vi "Parse Data Packet for Writing.vi"(10 "First Log Value in":bool, 11 "WiBCI16T Data in":T1 {"Reg Map"."ADS2" format="%x"; "Reg Map"."ADS1" format="%x"}) -> (3 "Array":dbl[](array[numeric]))   [LabVIEW 2016, in "Logger.lvlib"]
uses:
  Logger.lvlib
  Acquisition/WiBCI16T_Data.ctl
  Acquisition/WiBCI16T_Status.ctl
  Acquisition/Reg_Map.ctl
  Acquisition/Acquisition.lvlib
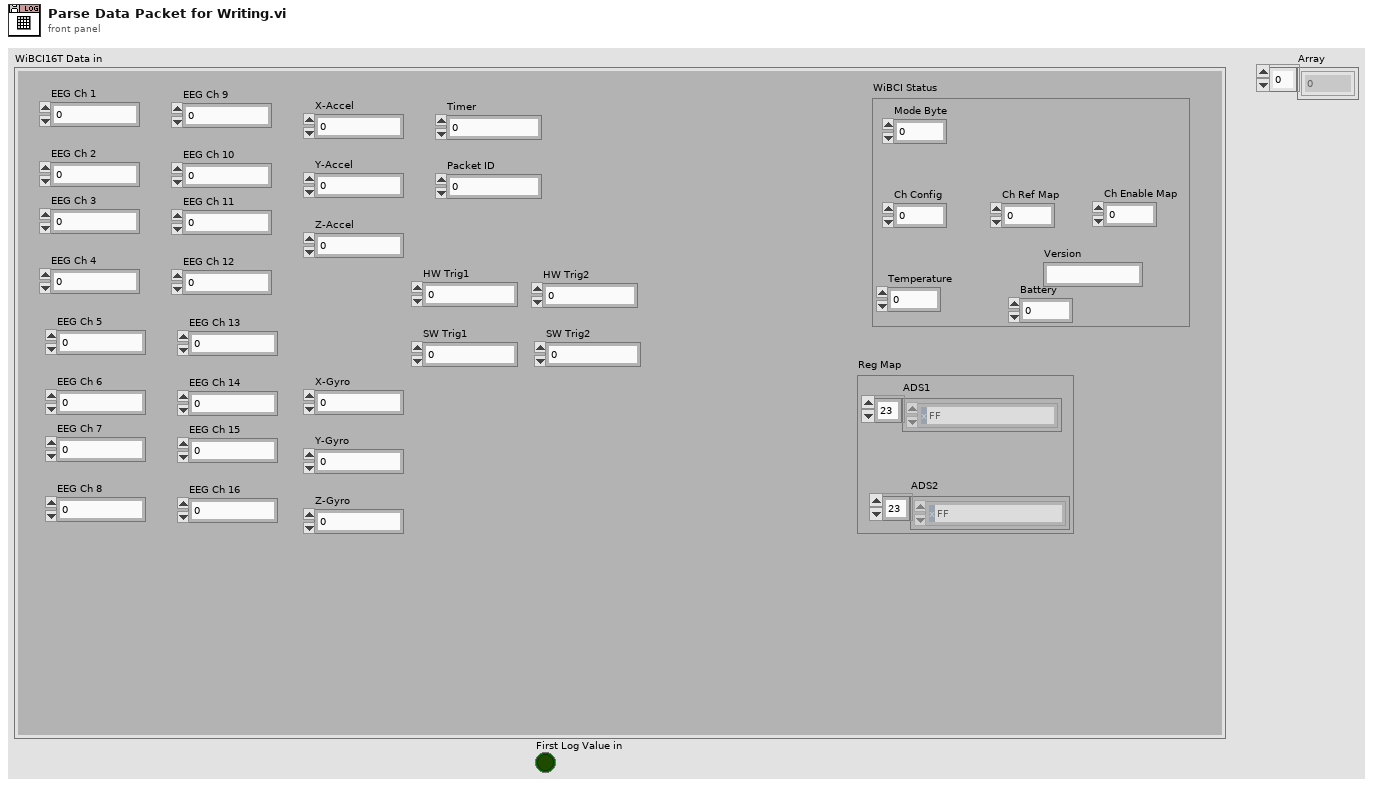
[diagram p1: front panel]
types:
  T1 = typedef "Acquisition.lvlib/WiBCI16T_Data.ctl" = cluster{"EEG Ch 1":dbl, "EEG Ch 2":dbl, "EEG Ch 3":dbl, "EEG Ch 4":dbl, "EEG Ch 5":dbl, "EEG Ch 6":dbl, "EEG Ch 7":dbl, "EEG Ch 8":dbl, "EEG Ch 9":dbl, "EEG Ch 10":dbl, "EEG Ch 11":dbl, "EEG Ch 12":dbl, "EEG Ch 13":dbl, "EEG Ch 14":dbl, "EEG Ch 15":dbl, "EEG Ch 16":dbl, "X-Accel":i16, "Y-Accel":i16, "Z-Accel":i16, "X-Gyro":i16, "Y-Gyro":i16, "Z-Gyro":i16, "Timer":u32, "Packet ID":u32, "HW Trig1":u8, "SW Trig1":i8, "HW Trig2":u8, "SW Trig2":i8, "WiBCI Status":T2, "Reg Map":T3}
  T2 = typedef "Acquisition.lvlib/WiBCI16T_Status.ctl" = cluster{"Mode Byte":u8, "Ch Config":u8, "Ch Ref Map":u16, "Ch Enable Map":u16, "Temperature":sgl, "Battery":u8, "Version":string}
  T3 = typedef "Acquisition.lvlib/Reg_Map.ctl" = cluster{"ADS1":u8[], "ADS2":u8[]}
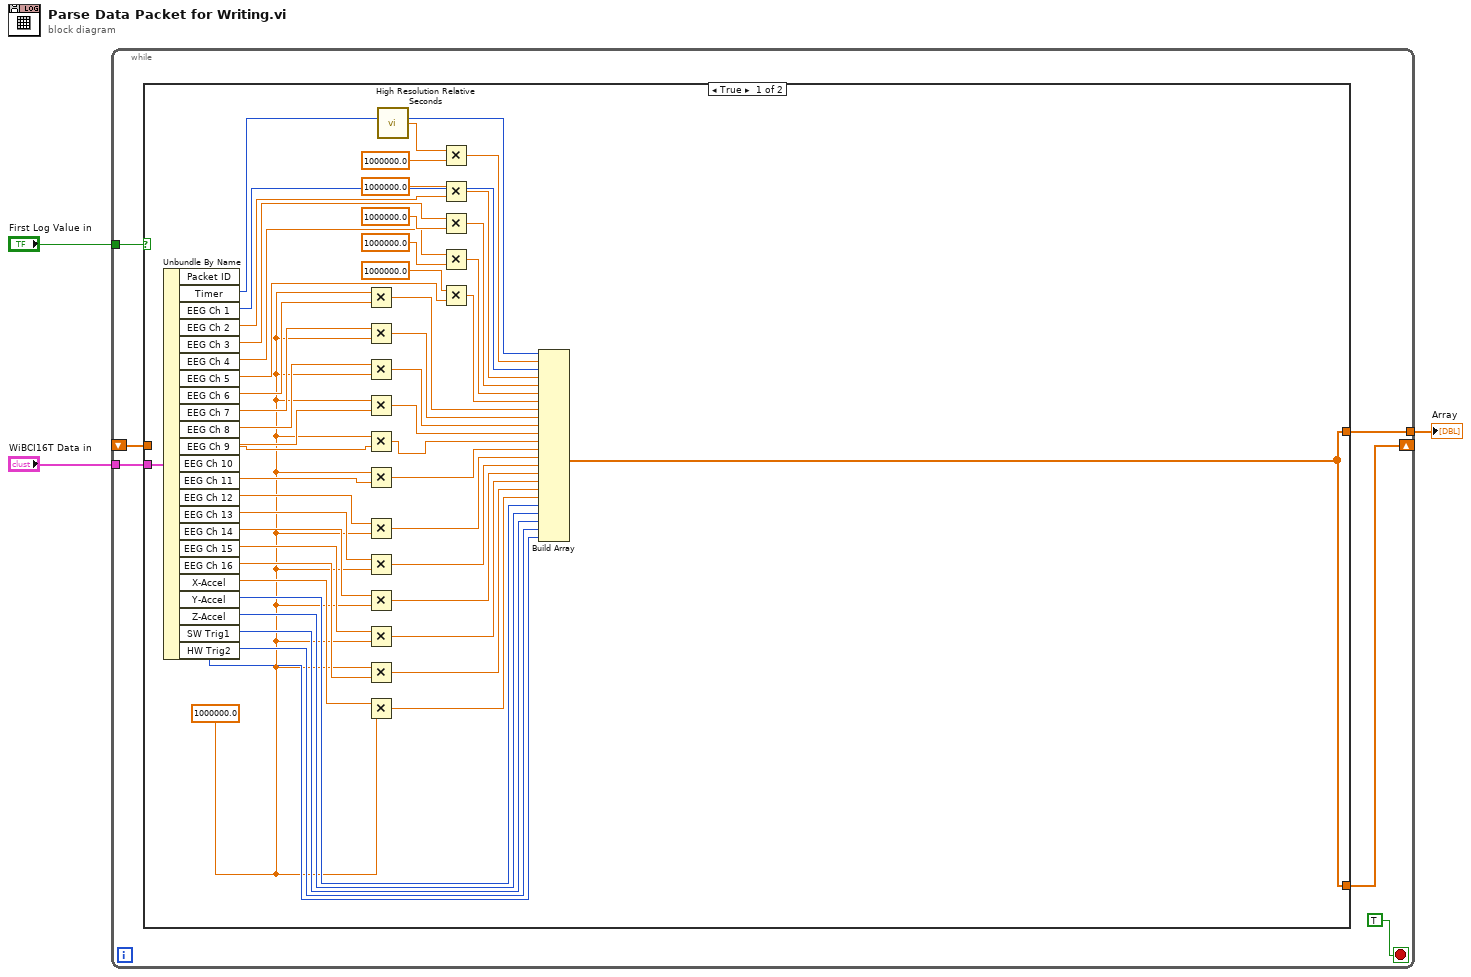
[diagram p0: block diagram]
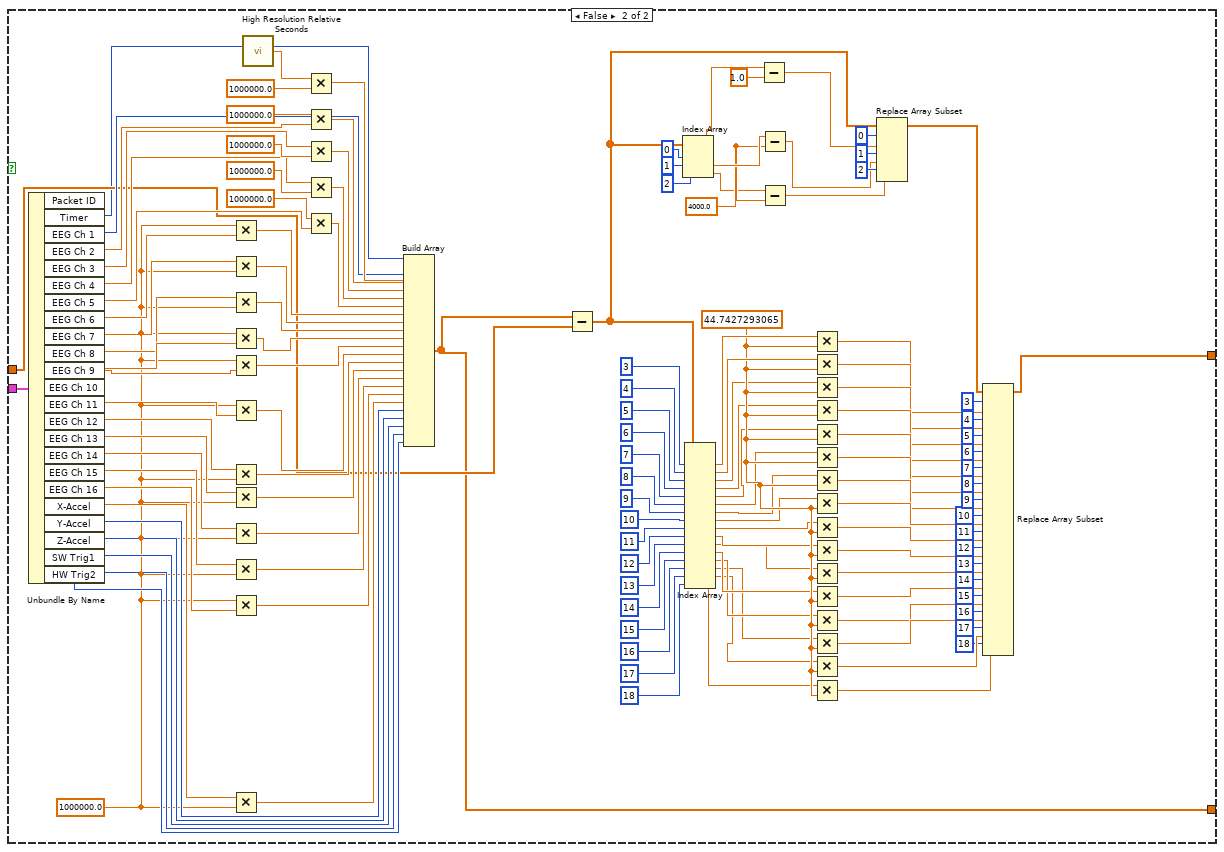
[diagram p2: hidden frame]
diagram:
  n1 = while {
    tunnel: [w9] -> w3
    shift-right: [w5] -> _
    shift-left: _ -> [w8]
    tunnel: "First Log Value in" -> [w6]
    tunnel: "WiBCI16T Data in" -> [w4]
    stop <- TRUE stop-if-true
    n2 = case shown="True" w6 {
      tunnel: [w10 w75] -> w9
      tunnel: w8 -> [_ w143]
      tunnel: [w10 w142] -> w5
      tunnel: w4 -> [w11 w144]
      frame True {
        w12 = 1000000.0 ("x")
        n3 = Unbundle By Name(w11) -> ("Packet ID"=w29:u32, "Timer"=w31:u32, "EEG Ch 1"=w32:dbl, "EEG Ch 2"=w33:dbl, "EEG Ch 3"=w34:dbl, "EEG Ch 4"=w35:dbl, "EEG Ch 5"=w36:dbl, "EEG Ch 6"=w37:dbl, "EEG Ch 7"=w38:dbl, "EEG Ch 8"=w39:dbl, "EEG Ch 9"=w40:dbl, "EEG Ch 10"=w41:dbl, "EEG Ch 11"=w42:dbl, "EEG Ch 12"=w43:dbl, "EEG Ch 13"=w44:dbl, "EEG Ch 14"=w45:dbl, "EEG Ch 15"=w46:dbl, "EEG Ch 16"=w47:dbl, "X-Accel"=w48:i16, "Y-Accel"=w49:i16, "Z-Accel"=w50:i16, "SW Trig1"=w51:i8, "HW Trig2"=w52:u8)
        n4 = Multiply(x=w12, y=w36) -> (x*y=w24:dbl)
        n5 = Multiply(x=w37, y=w12) -> (x*y=w23:dbl)
        n6 = Multiply(x=w38, y=w12) -> (x*y=w22:dbl)
        n7 = Multiply(x=w12, y=w39) -> (x*y=w21:dbl)
        n8 = Multiply(x=w12, y=w40) -> (x*y=w20:dbl)
        n9 = Multiply(x=w12, y=w41) -> (x*y=w19:dbl)
        n10 = Multiply(x=w42, y=w12) -> (x*y=w18:dbl)
        n11 = Multiply(x=w43, y=w12) -> (x*y=w17:dbl)
        n12 = Multiply(x=w44, y=w12) -> (x*y=w16:dbl)
        n13 = Multiply(x=w45, y=w12) -> (x*y=w14:dbl)
        n14 = Multiply(x=w12, y=w46) -> (x*y=w15:dbl)
        n15 = Multiply(x=w47, y=w12) -> (x*y=w13:dbl)
        n16 = call <vilib>:"High Resolution Relative Seconds.vi"() -> ("relative seconds"=w30:dbl)
        n17 = Multiply(x=w30, y=1000000.0) -> (x*y=w53:dbl)
        n18 = Multiply(x=1000000.0, y=w32) -> (x*y=w55:dbl)
        n19 = Multiply(x=w33, y=1000000.0) -> (x*y=w57:dbl)
        n20 = Multiply(x=w34, y=1000000.0) -> (x*y=w28:dbl)
        n21 = Multiply(x=1000000.0, y=w35) -> (x*y=w26:dbl)
        n22 = Build Array(w29, w53, w31, w55, w57, w28, w26, w24, w23, w22, w21, w20, w19, w18, w17, w16, w14, w15, w13, w48, w49, w50, w51, w52) -> (w10:dbl[])
      }
      frame False {
        w108 = 44.7427293065
        w137 = 4000.0 ("y")
        w145 = 1000000.0 ("x")
        n23 = Unbundle By Name(w144) -> ("Packet ID"=w141:u32, "Timer"=w163:u32, "EEG Ch 1"=w164:dbl, "EEG Ch 2"=w165:dbl, "EEG Ch 3"=w166:dbl, "EEG Ch 4"=w167:dbl, "EEG Ch 5"=w168:dbl, "EEG Ch 6"=w169:dbl, "EEG Ch 7"=w170:dbl, "EEG Ch 8"=w171:dbl, "EEG Ch 9"=w172:dbl, "EEG Ch 10"=w173:dbl, "EEG Ch 11"=w174:dbl, "EEG Ch 12"=w175:dbl, "EEG Ch 13"=w176:dbl, "EEG Ch 14"=w177:dbl, "EEG Ch 15"=w178:dbl, "EEG Ch 16"=w179:dbl, "X-Accel"=w180:i16, "Y-Accel"=w181:i16, "Z-Accel"=w182:i16, "SW Trig1"=w183:i8, "HW Trig2"=w184:u8)
        n24 = Multiply(x=w145, y=w168) -> (x*y=w157:dbl)
        n25 = Multiply(x=w169, y=w145) -> (x*y=w156:dbl)
        n26 = Multiply(x=w170, y=w145) -> (x*y=w155:dbl)
        n27 = Multiply(x=w145, y=w171) -> (x*y=w154:dbl)
        n28 = Multiply(x=w145, y=w172) -> (x*y=w153:dbl)
        n29 = Multiply(x=w145, y=w173) -> (x*y=w152:dbl)
        n30 = Multiply(x=w174, y=w145) -> (x*y=w151:dbl)
        n31 = Multiply(x=w175, y=w145) -> (x*y=w150:dbl)
        n32 = Multiply(x=w176, y=w145) -> (x*y=w149:dbl)
        n33 = Multiply(x=w177, y=w145) -> (x*y=w147:dbl)
        n34 = Multiply(x=w145, y=w178) -> (x*y=w148:dbl)
        n35 = Multiply(x=w179, y=w145) -> (x*y=w146:dbl)
        n36 = call <vilib>:"High Resolution Relative Seconds.vi"() -> ("relative seconds"=w162:dbl)
        n37 = Multiply(x=w162, y=1000000.0) -> (x*y=w185:dbl)
        n38 = Multiply(x=1000000.0, y=w164) -> (x*y=w187:dbl)
        n39 = Multiply(x=w165, y=1000000.0) -> (x*y=w189:dbl)
        n40 = Multiply(x=w166, y=1000000.0) -> (x*y=w161:dbl)
        n41 = Multiply(x=1000000.0, y=w167) -> (x*y=w159:dbl)
        n42 = Build Array(w141, w185, w163, w187, w189, w161, w159, w157, w156, w155, w154, w153, w152, w151, w150, w149, w147, w148, w146, w180, w181, w182, w183, w184) -> (w142:dbl[])
        n43 = Subtract(x=w142, y=w143) -> (x-y=w74:dbl[])
        n44 = Index Array(array=w74, index #1=0 ("index"), index #2=1 ("index"), index #3=2 ("index")) -> (element #1=w130:dbl, element #2=w138:dbl, element #3=w132:dbl)
        n45 = Index Array(array=w74, index #1=3 ("index"), index #2=4 ("index"), index #3=5 ("index"), index #4=6 ("index"), index #5=7 ("index"), index #6=8 ("index"), index #7=9 ("index"), index #8=10 ("index"), index #9=11 ("index"), index #10=12 ("index"), index #11=13 ("index"), index #12=14 ("index"), index #13=15 ("index"), index #14=16 ("index"), index #15=17 ("index"), index #16=18 ("index")) -> (element #1=w109:dbl, element #2=w110:dbl, element #3=w73:dbl, element #4=w72:dbl, element #5=w71:dbl, element #6=w70:dbl, element #7=w69:dbl, element #8=w68:dbl, element #9=w67:dbl, element #10=w66:dbl, element #11=w65:dbl, element #12=w64:dbl, element #13=w63:dbl, element #14=w62:dbl, element #15=w61:dbl, element #16=w60:dbl)
        n46 = Subtract(x=w130, y=1.0) -> (x-y=w127:dbl)
        n47 = Subtract(x=w138, y=w137) -> (x-y=w134:dbl)
        n48 = Subtract(x=w132, y=w137) -> (x-y=w133:dbl)
        n49 = Multiply(x=w109, y=w108) -> (x*y=w111:dbl)
        n50 = Multiply(x=w110, y=w108) -> (x*y=w112:dbl)
        n51 = Multiply(x=w73, y=w108) -> (x*y=w113:dbl)
        n52 = Multiply(x=w72, y=w108) -> (x*y=w114:dbl)
        n53 = Multiply(x=w71, y=w108) -> (x*y=w115:dbl)
        n54 = Multiply(x=w70, y=w108) -> (x*y=w116:dbl)
        n55 = Multiply(x=w69, y=w108) -> (x*y=w117:dbl)
        n56 = Multiply(x=w68, y=w108) -> (x*y=w118:dbl)
        n57 = Multiply(x=w67, y=w108) -> (x*y=w119:dbl)
        n58 = Multiply(x=w66, y=w108) -> (x*y=w120:dbl)
        n59 = Multiply(x=w65, y=w108) -> (x*y=w121:dbl)
        n60 = Multiply(x=w64, y=w108) -> (x*y=w122:dbl)
        n61 = Multiply(x=w63, y=w108) -> (x*y=w123:dbl)
        n62 = Multiply(x=w62, y=w108) -> (x*y=w124:dbl)
        n63 = Multiply(x=w61, y=w108) -> (x*y=w125:dbl)
        n64 = Multiply(x=w60, y=w108) -> (x*y=w126:dbl)
        n65 = Replace Array Subset(array=w74, new element #1=w127, index #1=0 ("index"), new element #2=w134, index #2=1 ("index"), new element #3=w133, index #3=2 ("index")) -> (w59:dbl[])
        n66 = Replace Array Subset(array=w59, new element #1=w111, index #1=3 ("index"), new element #2=w112, index #2=4 ("index"), new element #3=w113, index #3=5 ("index"), new element #4=w114, index #4=6 ("index"), new element #5=w115, index #5=7 ("index"), new element #6=w116, index #6=8 ("index"), new element #7=w117, index #7=9 ("index"), new element #8=w118, index #8=10 ("index"), new element #9=w119, index #9=11 ("index"), new element #10=w120, index #10=12 ("index"), new element #11=w121, index #11=13 ("index"), new element #12=w122, index #12=14 ("index"), new element #13=w123, index #13=15 ("index"), new element #14=w124, index #14=16 ("index"), new element #15=w125, index #15=17 ("index"), new element #16=w126, index #16=18 ("index")) -> (w75:dbl[])
      }
    }
  }
  "Array" <- w3
